vi "WPI_IMU_ADIS16448_Open.vi"(8 "error in":errorcluster, 9 "AHRS Algorithm":enum16{"Complementary", "Madgwick"}(ring), 10 "Yaw Axis":enum16{"X", "Y", "Z"}(ring)=enum."Z", 11 "SPI Chip Select":T3=enum."SPI MXP") -> (0 "error out":errorcluster, 3 "ADI IMU Interrupt DevRef":T1={"ADI IMU DevRef"={"DevStatus"={"status"=FALSE, "code"=0, "source"=""}, "Handle"=0, "SPI Bus"=enum."SPI On-Board, CS0", "Device Found"=FALSE, "Device Ready"=FALSE, "Yaw Axis"=enum."Z", "AHRS Algorithm"=enum."Complementary", "Serial"=0, "Lot ID 2"=0, "Lot ID 1"=0, "Product ID"=0}, "InterruptRef"={"DevStatus"={"status"=FALSE, "code"=0, "source"=""}, "InterruptIndex"=enum."0"}})   [LabVIEW 2015, in "Apple Pi Gyro Library.lvlib" / "FRC_ADIS16448_IMU.lvlib"]
doc: "Initiates communication between an Analog Devices MXP IMU and the RoboRIO."
uses:
  FRC_ADIS16448_IMU.lvlib
  <vilib>/Rock Robotics/SystemInterfaces/spilib/spi_bus.ctl
  WPI_IMU_ADIS16448_InterruptDevRef.ctl
  WPI_IMU_ADIS16448_IMUDevRef.ctl
  <vilib>/Rock Robotics/WPI/Interrupt/WPI_InterruptRef.ctl
  <vilib>/Rock Robotics/SystemInterfaces/Interrupt/FPGA_InterruptIndex.ctl
  <vilib>/Rock Robotics/WPI/SPI/WPI_SPIMode.ctl
  <vilib>/Rock Robotics/SystemInterfaces/DIO/FPGA_DIOChannel.ctl
  WPI_IMU_ADIS16448_Registers.ctl
  <vilib>/Rock Robotics/WPI/Counter/WPI_CounterDigitalInputToDigitalSource.vi
  <vilib>/Rock Robotics/SystemInterfaces/CounterEncoderSourceConvertion/FPGA_CounterEncoderSourceConvertionLVSourceTypeToFPGAType.vi
  <vilib>/Rock Robotics/WPI/Interrupt/WPI_InterruptCache.vi
  <vilib>/Rock Robotics/SystemInterfaces/Interrupt/FPGA_InterruptWriteConfiguration.vi
  <vilib>/Rock Robotics/SystemInterfaces/NetworkCommunication/NetComm_UsageReport_ResourceType.ctl
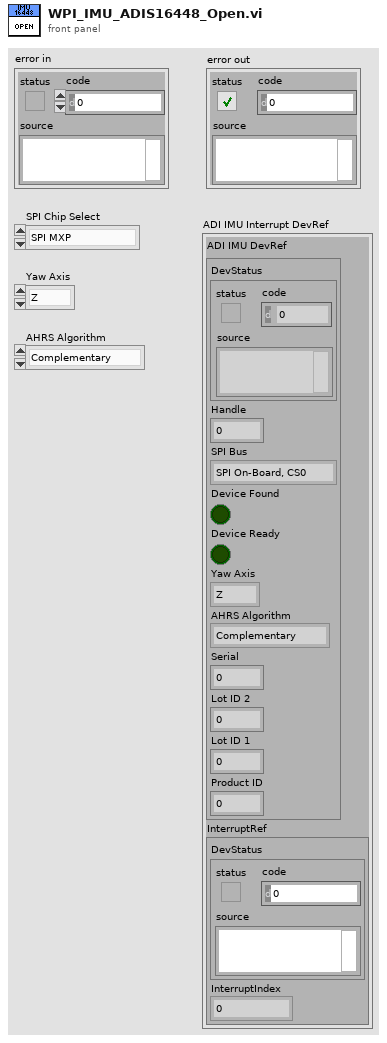
[diagram p1: front panel]
types:
  T1 = typedef "Apple Pi Gyro Library.lvlib/FRC_ADIS16448_IMU.lvlib/WPI_IMU_ADIS16448_InterruptDevRef.ctl" = cluster{"ADI IMU DevRef":T2, "InterruptRef":T4}
  T2 = typedef "Apple Pi Gyro Library.lvlib/FRC_ADIS16448_IMU.lvlib/WPI_IMU_ADIS16448_IMUDevRef.ctl" = cluster{"DevStatus":errorcluster, "Handle":i32, "SPI Bus":T3, "Device Found":bool, "Device Ready":bool, "Yaw Axis":enum16{"X", "Y", "Z"}, "AHRS Algorithm":enum16{"Complementary", "Madgwick"}, "Serial":u16, "Lot ID 2":u16, "Lot ID 1":u16, "Product ID":u16}
  T3 = typedef "spi_bus.ctl" = enum16{"SPI On-Board, CS0", "SPI On-Board, CS1", "SPI On-Board, CS2", "SPI On-Board, CS3", "SPI MXP", "Invalid"}
  T4 = typedef "WPI_InterruptRef.ctl" = cluster{"DevStatus":errorcluster, "InterruptIndex":T5}
  T5 = typedef "FPGA_InterruptIndex.ctl" = enum8{"0", "1", "2", "3", "4", "5", "6", "7", "Invalid"}
  T6 = typedef "FPGA_DIOChannel.ctl" = enum8{"DIO 0", "DIO 1", "DIO 2", "DIO 3", "DIO 4", "DIO 5", "DIO 6", "DIO 7", "DIO 8", "DIO 9", "DIO MXP 0", "DIO MXP 1", "DIO MXP 2", "DIO MXP 3", "DIO MXP 4", "DIO MXP 5", "DIO MXP 6", "DIO MXP 7", "DIO MXP 8", "DIO MXP 9", "DIO MXP 10", "DIO MXP 11", "DIO MXP 12", "DIO MXP 13", "DIO MXP 14", "DIO MXP 15", "Invalid"}
  T7 = typedef "WPI_SPIMode.ctl" = enum16{"Mode 0 (Clk Idle Low,Sample on Leading)", "Mode 1 (Clk Idle Low,Sample on Trailing)", "Mode 2 (Clk Idle High,Sample on Leading)", "Mode 3 (Clk Idle High,Sample on Trailing)"}
  T8 = typedef "Apple Pi Gyro Library.lvlib/FRC_ADIS16448_IMU.lvlib/WPI_IMU_ADIS16448_Registers.ctl" = u8
  T9 = typedef "WPI_DigitalOutputDevRef.ctl" = cluster{"DIO Channel":T6, "DevStatus":errorcluster}
  T10 = typedef "WPI_DigitalInputDevRef.ctl" = cluster{"DevStatus":errorcluster, "DIO Channel":T6}
  T11 = typedef "WPI_SPIDevRef.ctl" = cluster{"DevStatus":errorcluster, "Handle":i32, "SPI Bus":T3}
  T12 = typedef "FPGA_CounterEncoderSourceConvertionLVSourceType.ctl" = cluster{"DevStatus":errorcluster, "AnalogTriggerMode?":bool, "DigitalMode":cluster{"DIO Channel":T13}, "AnalogTriggerMode":cluster{"AnalogTriggerIndex":T14, "OutputType":T15}}
  T13 = typedef "FPGA_DIODigitalSourceChannel.ctl" = enum8{"DIO 0", "DIO 1", "DIO 2", "DIO 3", "DIO 4", "DIO 5", "DIO 6", "DIO 7", "DIO 8", "DIO 9", "DIO MXP 0", "DIO MXP 1", "DIO MXP 2", "DIO MXP 3", "DIO MXP 4", "DIO MXP 5", "DIO MXP 6", "DIO MXP 7", "DIO MXP 8", "DIO MXP 9", "DIO MXP 10", "DIO MXP 11", "DIO MXP 12", "DIO MXP 13", "DIO MXP 14", "DIO MXP 15", "Disabled"}
  T14 = typedef "FPGA_AnalogTriggerIndex.ctl" = enum8{"Trig 0", "Trig 1", "Trig 2", "Trig 3", "Trig 4", "Trig 5", "Trig 6", "Trig 7", "Invalid"}
  T15 = typedef "FPGA_AnalogTriggerOutType.ctl" = enum16{"InWindow", "TriggerState", "Rising", "Falling"}
  T16 = typedef "NetComm_UsageReport_ResourceType.ctl" = enum8{"Controller", "Module", "Language", "CANPlugin", "Accelerometer", "ADXL345", "AnalogChannel", "AnalogTrigger", "AnalogTriggerOutput", "CANJaguar", "Compressor", "Counter", "Dashboard", "DigitalInput", "DigitalOutput", "DriverStationCIO", "DriverStationEIO", "DriverStationLCD", "Encoder", "GearTooth", "Gyro", "I2C", "Framework", "Jaguar", "Joystick", "Kinect", "KinectStick", "PIDController", "Preferences", "PWM", "Relay", "RobotDrive", "SerialPort", "Servo", "Solenoid", "SPI", "Task", "Ultrasonic", "Victor", "Button", "Command", "AxisCamera", "PCVideoServer", "SmartDashboard", "Talon", "HiTechnicColorSensor", "HiTechnicAccel", "HiTechnicCompass", "SRF08", "AnalogOutput", "Victor SP", "Talon SRX", "CAN Talon SRX", "ADXL362 Accel", "ADXRS450 Gyro", "Rev SPARK", "Mindsensors SD540", "Digital Filter", "ADIS16448"}
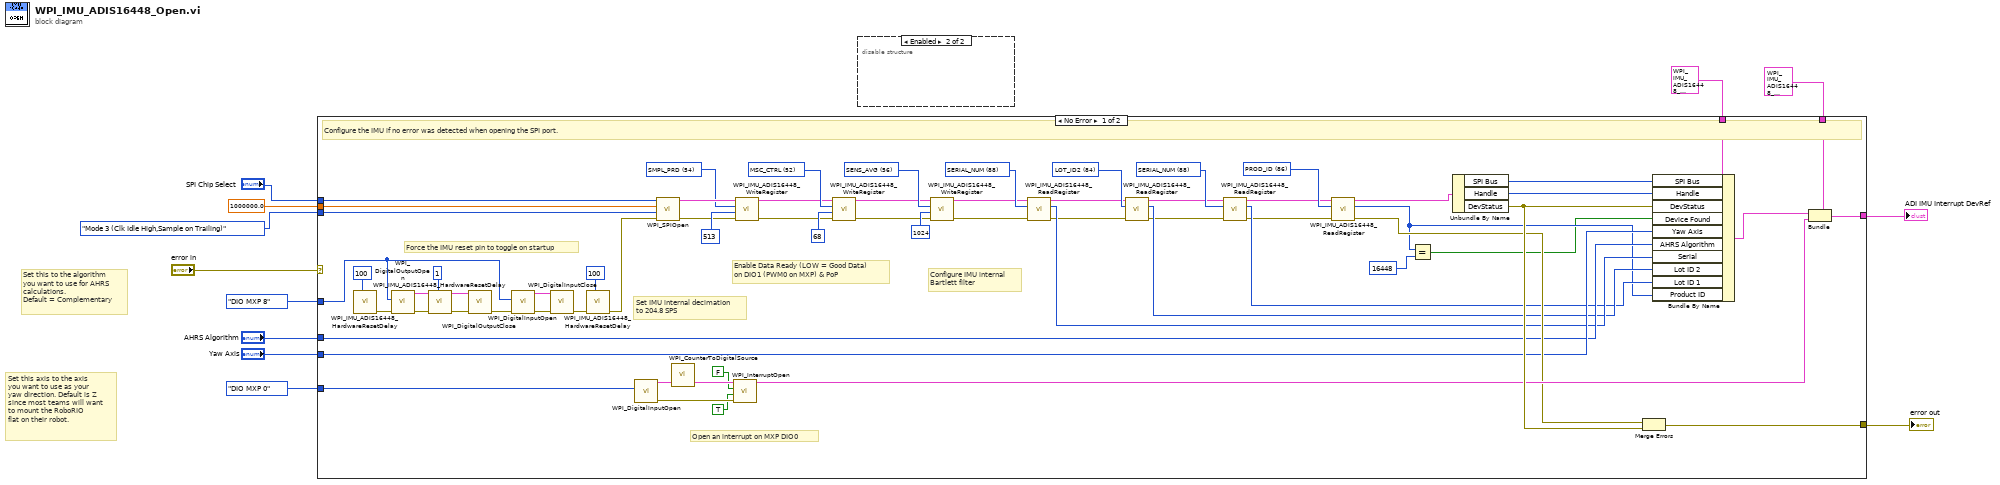
[diagram p0: block diagram]
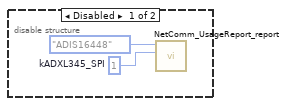
[diagram p2: hidden frame]
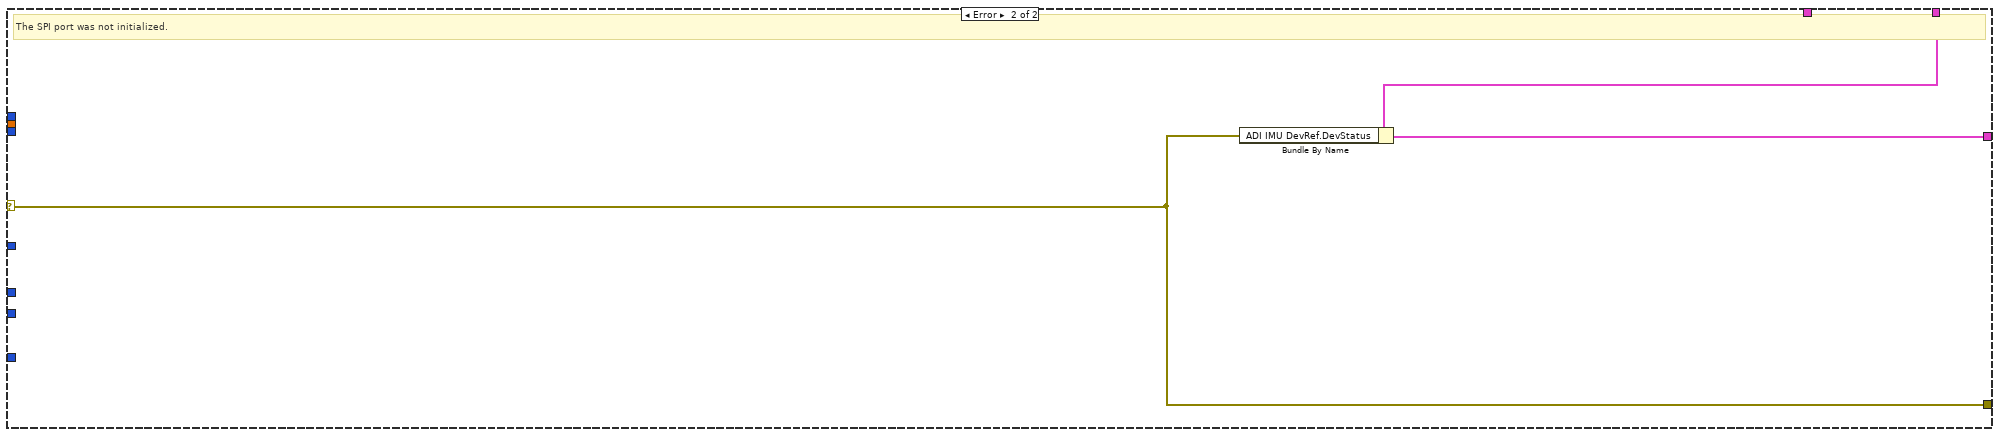
[diagram p3: hidden frame]
diagram:
  # "Set this to the algorithm\nyou want to use for AHRS\ncalculations. \nDefault = Complementary"
  # "Set this axis to the axis\nyou want to use as your\nyaw direction. Default is Z\nsince most teams will want \nto mount the RoboRIO\nflat on their robot."
  n1 = case shown="No Error" "error in" {
    selector: "error in" -> [_ w80]
    tunnel: "SPI Chip Select" -> [w78 _]
    tunnel: 1000000.0 ("Clock Rate (Hz)") -> [w77 _]
    tunnel: WPI_SPIMode."Mode 3 (Clk Idle High,Sample on Trailing)" ("Mode (3)") -> [w76 _]
    tunnel: [w70 w80] -> w8
    tunnel: T2 {"DevStatus"={"status"=FALSE, "code"=0, "source"=""}, "Handle"=0, "SPI Bus"=enum."SPI On-Board, CS0", "Device Found"=FALSE, "Device Ready"=FALSE, "Yaw Axis"=enum."Z", "AHRS Algorithm"=enum."Complementary", "Serial"=0, "Lot ID 2"=0, "Lot ID 1"=0, "Product ID"=0} ("SimpleGyroDevRef 2") -> [w75 _]
    tunnel: [w61 w79] -> w1
    tunnel: T1 {"ADI IMU DevRef"={"DevStatus"={"status"=FALSE, "code"=0, "source"=""}, "Handle"=0, "SPI Bus"=enum."SPI On-Board, CS0", "Device Found"=FALSE, "Device Ready"=FALSE, "Yaw Axis"=enum."Z", "AHRS Algorithm"=enum."Complementary", "Serial"=0, "Lot ID 2"=0, "Lot ID 1"=0, "Product ID"=0}, "InterruptRef"={"DevStatus"={"status"=FALSE, "code"=0, "source"=""}, "InterruptIndex"=enum."0"}} ("output cluster") -> [w60 w81]
    tunnel: FPGA_DIOChannel."DIO MXP 0" ("DIO Channel") -> [w59 _]
    tunnel: "Yaw Axis" -> [w54 _]
    tunnel: "AHRS Algorithm" -> [w53 _]
    tunnel: FPGA_DIOChannel."DIO MXP 8" ("DIO Channel") -> [w15 _]
    frame No Error {
      w33 = T8 86 items=["GLOB_CMD"=62, "SEQ_CNT"=58, "SMPL_PRD"=54, "SENS_AVG"=56, "MSC_CTRL"=52, "ERROR_FLAGS"=60, "TEMP"=44, "BARO"=40, "Z_MAG"=36, "Y_MAG"=32, "X_MAG"=28, "Z_ACCEL"=24, "Y_ACCEL"=20, "X_ACCEL"=16, "Z_GYRO"=12, "Y_GYRO"=8, "X_GYRO"=4, "PROD_ID"=86, "LOT_ID2"=84, "LOT_ID1"=82, "SERIAL_NUM"=88] ("ADIS16448 Register")
      w34 = T8 88 items=["GLOB_CMD"=62, "SEQ_CNT"=58, "SMPL_PRD"=54, "SENS_AVG"=56, "MSC_CTRL"=52, "ERROR_FLAGS"=60, "TEMP"=44, "BARO"=40, "Z_MAG"=36, "Y_MAG"=32, "X_MAG"=28, "Z_ACCEL"=24, "Y_ACCEL"=20, "X_ACCEL"=16, "Z_GYRO"=12, "Y_GYRO"=8, "X_GYRO"=4, "PROD_ID"=86, "LOT_ID2"=84, "LOT_ID1"=82, "SERIAL_NUM"=88] ("ADIS16448 Register")
      w36 = T8 84 items=["GLOB_CMD"=62, "SEQ_CNT"=58, "SMPL_PRD"=54, "SENS_AVG"=56, "MSC_CTRL"=52, "ERROR_FLAGS"=60, "TEMP"=44, "BARO"=40, "Z_MAG"=36, "Y_MAG"=32, "X_MAG"=28, "Z_ACCEL"=24, "Y_ACCEL"=20, "X_ACCEL"=16, "Z_GYRO"=12, "Y_GYRO"=8, "X_GYRO"=4, "PROD_ID"=86, "LOT_ID2"=84, "LOT_ID1"=82, "SERIAL_NUM"=88] ("ADIS16448 Register")
      w39 = T8 88 items=["GLOB_CMD"=62, "SEQ_CNT"=58, "SMPL_PRD"=54, "SENS_AVG"=56, "MSC_CTRL"=52, "ERROR_FLAGS"=60, "TEMP"=44, "BARO"=40, "Z_MAG"=36, "Y_MAG"=32, "X_MAG"=28, "Z_ACCEL"=24, "Y_ACCEL"=20, "X_ACCEL"=16, "Z_GYRO"=12, "Y_GYRO"=8, "X_GYRO"=4, "PROD_ID"=86, "LOT_ID2"=84, "LOT_ID1"=82, "SERIAL_NUM"=88] ("ADIS16448 Register")
      w40 = T8 56 items=["GLOB_CMD"=62, "SEQ_CNT"=58, "SMPL_PRD"=54, "SENS_AVG"=56, "MSC_CTRL"=52, "ERROR_FLAGS"=60, "TEMP"=44, "BARO"=40, "Z_MAG"=36, "Y_MAG"=32, "X_MAG"=28, "Z_ACCEL"=24, "Y_ACCEL"=20, "X_ACCEL"=16, "Z_GYRO"=12, "Y_GYRO"=8, "X_GYRO"=4, "PROD_ID"=86, "LOT_ID2"=84, "LOT_ID1"=82, "SERIAL_NUM"=88] ("ADIS16448 Register")
      w41 = T8 52 items=["GLOB_CMD"=62, "SEQ_CNT"=58, "SMPL_PRD"=54, "SENS_AVG"=56, "MSC_CTRL"=52, "ERROR_FLAGS"=60, "TEMP"=44, "BARO"=40, "Z_MAG"=36, "Y_MAG"=32, "X_MAG"=28, "Z_ACCEL"=24, "Y_ACCEL"=20, "X_ACCEL"=16, "Z_GYRO"=12, "Y_GYRO"=8, "X_GYRO"=4, "PROD_ID"=86, "LOT_ID2"=84, "LOT_ID1"=82, "SERIAL_NUM"=88] ("ADIS16448 Register")
      w42 = T8 54 items=["GLOB_CMD"=62, "SEQ_CNT"=58, "SMPL_PRD"=54, "SENS_AVG"=56, "MSC_CTRL"=52, "ERROR_FLAGS"=60, "TEMP"=44, "BARO"=40, "Z_MAG"=36, "Y_MAG"=32, "X_MAG"=28, "Z_ACCEL"=24, "Y_ACCEL"=20, "X_ACCEL"=16, "Z_GYRO"=12, "Y_GYRO"=8, "X_GYRO"=4, "PROD_ID"=86, "LOT_ID2"=84, "LOT_ID1"=82, "SERIAL_NUM"=88] ("ADIS16448 Register")
      # "Force the IMU reset pin to toggle on startup"
      # "Open an interrupt on MXP DIO0"
      # "Configure IMU internal\nBartlett filter"
      # "Enable Data Ready (LOW = Good Data) \non DIO1 (PWM0 on MXP) & PoP"
      # "Set IMU internal decimation\nto 204.8 SPS"
      # "Configure the IMU if no error was detected when opening the SPI port."
      n2 = call "WPI_IMU_ADIS16448_HardwareResetDelay.vi"("Delay (ms)"=u32 100) -> ("error out"=w16:errorcluster)  [unwired: 9 in, 1 out]
      n3 = call <vilib>:"WPI_DigitalOutputOpen.vi"("error in (no error)"=w16, "DIO Channel"=w15) -> ("error out"=w46:errorcluster, "DigitalOutputDevRef"=w47:T9)  [unwired: 8 in]
      n4 = call "WPI_IMU_ADIS16448_HardwareResetDelay.vi"("Delay (ms)"=u32 1, "error in"=w46, "DigitalOutputDevRef"=w47) -> ("error out"=w49:errorcluster, "DigitalOutputDevRef"=w48:T9)  [unwired: 7 in]
      n5 = call <vilib>:"WPI_DigitalOutputClose.vi"("error in (no error)"=w49, "DigitalOutputDevRef"=w48) -> ("error out"=w45:errorcluster)  [unwired: 9 in]
      n6 = call <vilib>:"WPI_DigitalInputOpen.vi"("error in (no error)"=w45, "DIO Channel"=w15) -> ("error out"=w44:errorcluster, "DigitalInputDevRef"=w43:T10)  [unwired: 8 in]
      n7 = call <vilib>:"WPI_DigitalInputClose.vi"("error in (no error)"=w44, "DigitalInputDevRef"=w43) -> ("error out"=w31:errorcluster)  [unwired: 9 in]
      n8 = call "WPI_IMU_ADIS16448_HardwareResetDelay.vi"("Delay (ms)"=u32 100, "error in"=w31) -> ("error out"=w30:errorcluster)  [unwired: 8 in, 1 out]
      n9 = call <vilib>:"WPI_DigitalInputOpen.vi"("DIO Channel"=w59) -> ("error out"=w66:errorcluster, "DigitalInputDevRef"=w68:T10)  [unwired: 9 in]
      n10 = call <vilib>:"WPI_SPIOpen.vi"("error in"=w30, "Mode (3)"=w76, "Clock Rate (Hz)"=w77, "SPI Bus"=w78) -> ("error out"=w50:errorcluster, "SPIDevRef"=w51:T11)  [unwired: 6 in]
      n11 = call-poly <vilib>:"WPI_CounterToDigitalSource.vi"("DigitalInputDevRef"=w68) -> ("Digital Source"=w67:T12)  [unwired: 6 in]
      n12 = call <vilib>:"WPI_InterruptOpen.vi"("error in (no error)"=w66, "Falling Edge"=TRUE, "Rising Edge"=FALSE, "Source"=w67) -> ("InterruptRef"=w63:T4)  [unwired: 6 in, 1 out]
      n13 = call "WPI_IMU_ADIS16448_WriteRegister.vi"("error in (no error)"=w50, "Data"=u16 513, "ADIS16448 Register"=w42, "SPIDevRef in"=w51) -> ("error out"=w27:errorcluster, "SPIDevRef out"=w28:T11)  [unwired: 6 in]
      n14 = call "WPI_IMU_ADIS16448_WriteRegister.vi"("error in (no error)"=w27, "Data"=u16 68, "ADIS16448 Register"=w41, "SPIDevRef in"=w28) -> ("error out"=w25:errorcluster, "SPIDevRef out"=w26:T11)  [unwired: 6 in]
      n15 = call "WPI_IMU_ADIS16448_WriteRegister.vi"("error in (no error)"=w25, "Data"=u16 1024, "ADIS16448 Register"=w40, "SPIDevRef in"=w26) -> ("error out"=w23:errorcluster, "SPIDevRef out"=w24:T11)  [unwired: 6 in]
      n16 = call "WPI_IMU_ADIS16448_ReadRegister.vi"("error in (no error)"=w23, "ADIS16448 Register"=w39, "SPIDevRef in"=w24) -> ("error out"=w21:errorcluster, "Register Value"=w38:u16, "SPIDevRef out"=w22:T11)  [unwired: 6 in]
      n17 = call "WPI_IMU_ADIS16448_ReadRegister.vi"("error in (no error)"=w21, "ADIS16448 Register"=w36, "SPIDevRef in"=w22) -> ("error out"=w19:errorcluster, "Register Value"=w37:u16, "SPIDevRef out"=w20:T11)  [unwired: 6 in]
      n18 = call "WPI_IMU_ADIS16448_ReadRegister.vi"("error in (no error)"=w19, "ADIS16448 Register"=w34, "SPIDevRef in"=w20) -> ("error out"=w17:errorcluster, "Register Value"=w35:u16, "SPIDevRef out"=w18:T11)  [unwired: 6 in]
      n19 = call "WPI_IMU_ADIS16448_ReadRegister.vi"("error in (no error)"=w17, "ADIS16448 Register"=w33, "SPIDevRef in"=w18) -> ("error out"=w57:errorcluster, "Register Value"=w32:u16, "SPIDevRef out"=w58:T11)  [unwired: 6 in]
      n20 = Equal?(x=w32, y=u16 16448) -> (x = y?=w13:bool)
      n21 = Unbundle By Name(w58) -> ("SPI Bus"=w74:T3, "Handle"=w73:i32, "DevStatus"=w71:errorcluster)
      n22 = Merge Errors(w57, w71) -> (w70:errorcluster)
      n23 = Bundle By Name(cluster=w75, "SPI Bus"=w74, "Handle"=w73, "DevStatus"=w71, "Device Found"=w13, "Yaw Axis"=w54, "AHRS Algorithm"=w53, "Serial"=w38, "Lot ID 2"=w37, "Lot ID 1"=w35, "Product ID"=w32) -> (w62:T2)
      n24 = Bundle(cluster=w60, "ADI IMU DevRef"=w62, "InterruptRef"=w63) -> (w61:T1)
    }
    frame Error {
      # "The SPI port was not initialized."
      n25 = Bundle By Name(cluster=w81, "ADI IMU DevRef.DevStatus"=w80) -> (w79:T1)
    }
  }
  "error out" <- w8
  "ADI IMU Interrupt DevRef" <- w1
  n26 = disable-structure shown="Enabled" {
    frame Disabled {
      w83 = u8 1  # kADXL345_SPI
      n27 = call <vilib>:"NetComm_UsageReport_report.vi"("Instance Number"=w83, "Resource Type"=NetComm_UsageReport_ResourceType."ADIS16448") -> ()  [unwired: 10 in]
    }
    frame Enabled {
    }
  }
